vi "ReadHawkeyePathConfig.vi"(8 "error in (no error)":errorcluster, 11 "Workspace Path":path=path "E:/sw-deps-monitor") -> (0 "error out":errorcluster, 3 "Hawkeye Path Config Out":T1)   [LabVIEW 2019, in "Hawkeye.lvlib"]
uses:
  Hawkeye.lvlib
  Typedefs/HawkeyePathConfigs.ctl
  <userlib>/_OpenG.lib/file/file.llb/File Exists - Scalar__ogtk.vi
  <vilib>/Utility/config.llb/NI_LVConfig.lvlib
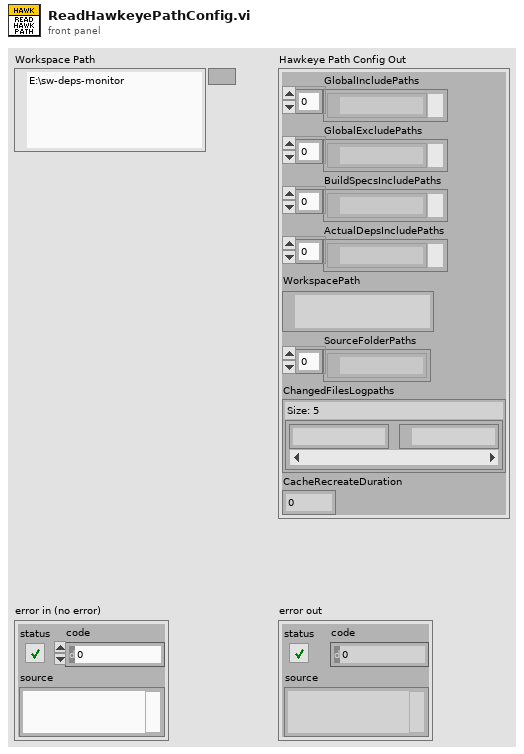
[diagram p1: front panel]
types:
  T1 = typedef "Hawkeye.lvlib/HawkeyePathConfigs.ctl" = cluster{"GlobalIncludePaths":path[], "GlobalExcludePaths":path[], "BuildSpecsIncludePaths":path[], "ActualDepsIncludePaths":path[], "WorkspacePath":path, "SourceFolderPaths":path[], "ChangedFilesLogpaths":map{string, path}, "CacheRecreateDuration":dbl}
  T2 = typedef "NI_LVConfig.lvlib/Config Data RefNum.ctl" = refnum<k1>
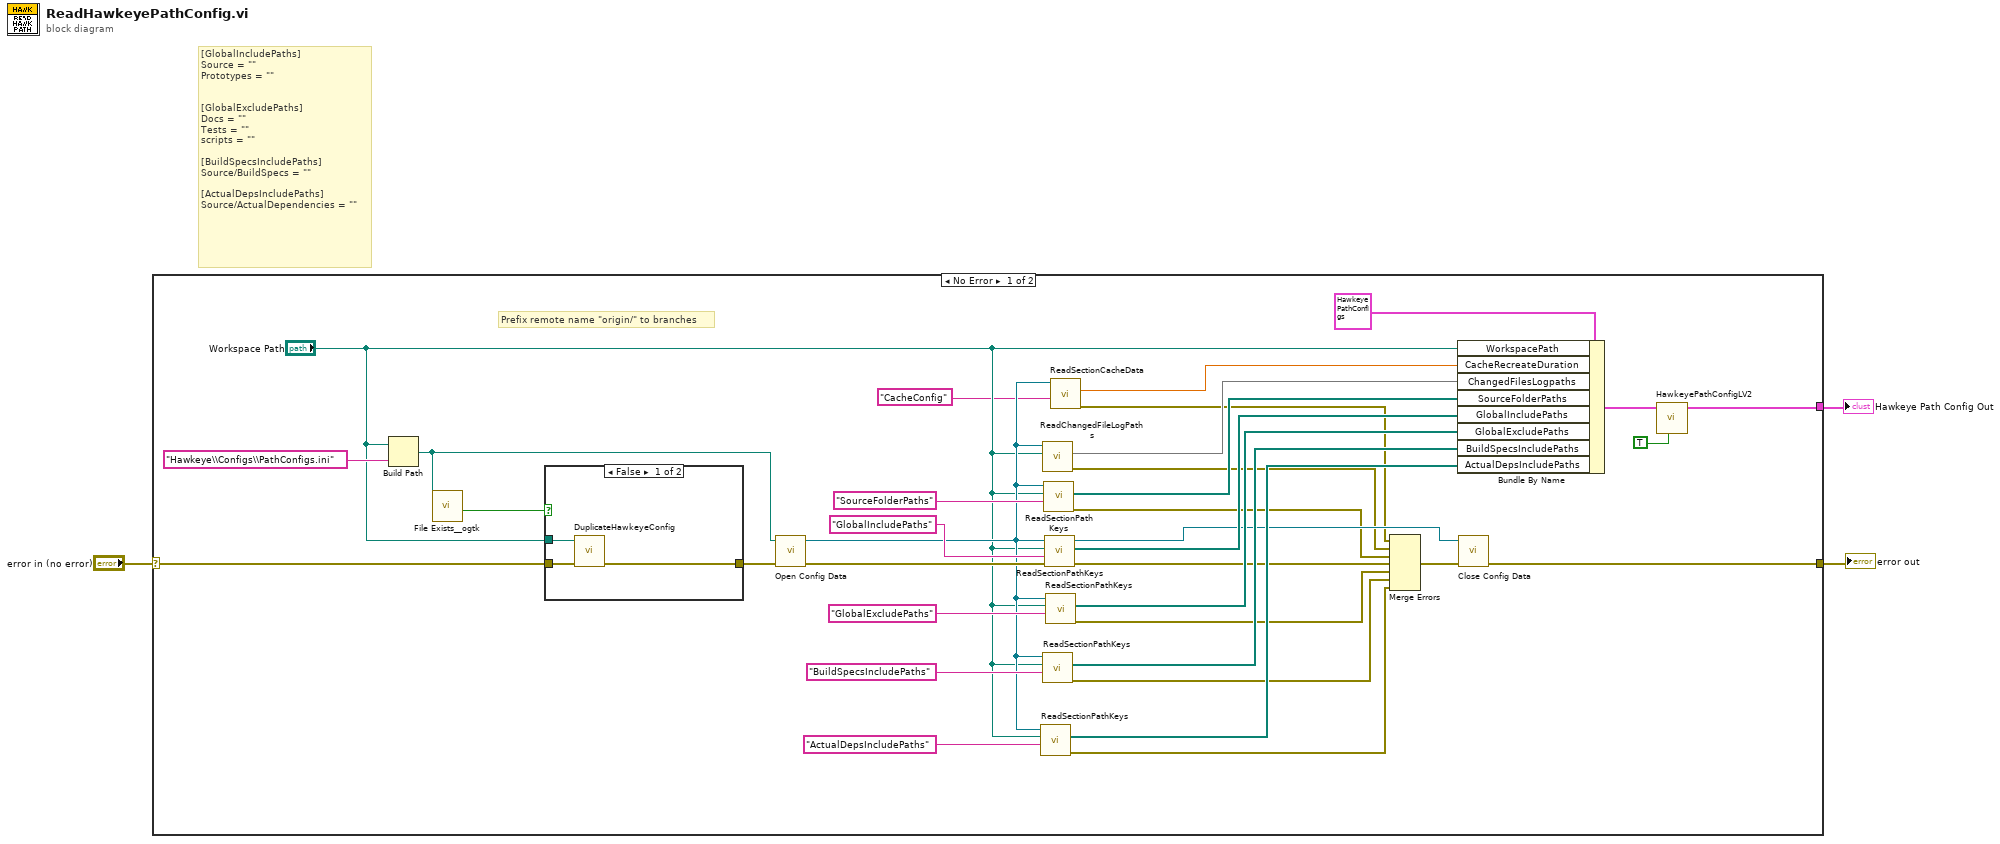
[diagram p0: block diagram]
diagram:
  # "[GlobalIncludePaths]\nSource = \"\"\nPrototypes = \"\"\n\n\n[GlobalExcludePaths]\nDocs = \"\"\nTests = \"\"\nscripts = \"\"\n\n[BuildSpecsIncludePaths]\nSource/BuildSpecs = \"\"\n\n[ActualDepsIncludePaths]\nSource/ActualDependencies = \"\""
  n1 = case shown="No Error" "error in (no error)" {
    selector: "error in (no error)" -> [w38 w43]
    tunnel: [w22 w43] -> w2
    tunnel: [w20 _] -> w1
    frame No Error {
      # "Prefix remote name \"origin/\" to branches"
      n2 = Build Path(base path="Workspace Path", name or relative path="Hawkeye\\Configs\\PathConfigs.ini" ("CICD Path Config Rel")) -> (appended path=w11:path)
      n3 = call-poly <userlib>:"File Exists__ogtk.vi"("file path"=w11) -> ("exists"=w14:bool)  [unwired: 6 in, 1 out]
      n4 = case shown="False" w14 {
        tunnel: w38 -> [w39 w42]
        tunnel: [w40 w42] -> w13
        tunnel: "Workspace Path" -> [w41 _]
        frame False {
          n5 = call "DuplicateHawkeyeConfig.vi"("error in (no error)"=w39, "Repo / Workspace Folder Path"=w41) -> ("error out"=w40:errorcluster)  [unwired: 9 in]
        }
        frame True {
        }
      }
      n6 = call <vilib>:"Open Config Data.vi"("error in (no error)"=w13, "configuration file path"=w11) -> ("error out"=w12:errorcluster, "refnum"=w8:T2)  [unwired: 7 in, 1 out]
      n7 = call "ReadSectionPathKeys.vi"("section"="ActualDepsIncludePaths", "Workspace Path"="Workspace Path", "Refnum in"=w8) -> ("error out"=w25:errorcluster, "Paths"=w29:path[])  [unwired: 6 in, 1 out]
      n8 = call "ReadChangedFileLogPaths.vi"("Workspace Path"="Workspace Path", "Refnum in"=w8) -> ("error out"=w15:errorcluster, "ChangedFilesLogpaths"=w16:map{string, path})  [unwired: 7 in, 1 out]
      n9 = call "ReadSectionPathKeys.vi"("section"="BuildSpecsIncludePaths", "Workspace Path"="Workspace Path", "Refnum in"=w8) -> ("error out"=w26:errorcluster, "Paths"=w30:path[])  [unwired: 6 in, 1 out]
      n10 = call "ReadSectionPathKeys.vi"("section"="SourceFolderPaths", "Workspace Path"="Workspace Path", "Refnum in"=w8) -> ("error out"=w18:errorcluster, "Paths"=w17:path[])  [unwired: 6 in, 1 out]
      n11 = call "ReadSectionPathKeys.vi"("error in (no error)"=w12, "section"="GlobalIncludePaths", "Workspace Path"="Workspace Path", "Refnum in"=w8) -> ("error out"=w28:errorcluster, "Paths"=w32:path[], "refnum out"=w23:T2)  [unwired: 5 in]
      n12 = call "ReadSectionPathKeys.vi"("section"="GlobalExcludePaths", "Workspace Path"="Workspace Path", "Refnum in"=w8) -> ("error out"=w27:errorcluster, "Paths"=w31:path[])  [unwired: 6 in, 1 out]
      n13 = call "ReadSectionCacheData.vi"("section"="CacheConfig", "Refnum in"=w8) -> ("error out"=w4:errorcluster, "CacheRecreateDuration"=w5:dbl)  [unwired: 7 in, 1 out]
      n14 = Merge Errors(w4, w15, w18, w28, w27, w26, w25) -> (w24:errorcluster)
      n15 = Bundle By Name(cluster=T1 {"GlobalIncludePaths"=[], "GlobalExcludePaths"=[], "BuildSpecsIncludePaths"=[], "ActualDepsIncludePaths"=[], "WorkspacePath"=path "", "SourceFolderPaths"=[], "ChangedFilesLogpaths"={}, "CacheRecreateDuration"=0.0}, "WorkspacePath"="Workspace Path", "CacheRecreateDuration"=w5, "ChangedFilesLogpaths"=w16, "SourceFolderPaths"=w17, "GlobalIncludePaths"=w32, "GlobalExcludePaths"=w31, "BuildSpecsIncludePaths"=w30, "ActualDepsIncludePaths"=w29) -> (w21:T1)
      n16 = call <vilib>:"Close Config Data.vi"("error in (no error)"=w24, "refnum"=w23) -> ("error out"=w22:errorcluster)  [unwired: 8 in, 1 out]
      n17 = call "HawkeyePathConfigLV2.vi"("Set? (F)"=TRUE, "Hawkeye Path Config In"=w21) -> ("Hawkeye Path Config Out"=w20:T1)  [unwired: 9 in]
    }
    frame Error {
    }
  }
  "error out" <- w2
  "Hawkeye Path Config Out" <- w1
